vi "Check for errors.vi"(8 "error in (no error)":errorcluster, 11 "System states in":T1) -> (0 "error out":errorcluster, 3 "System states out":T1)   [LabVIEW 2015]
uses:
  Type defs/System states.ctl
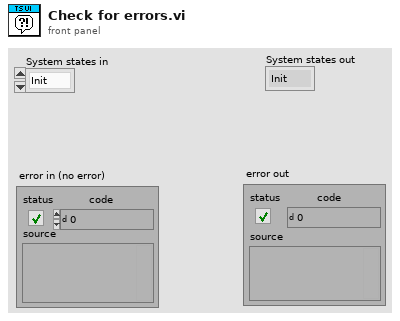
[diagram p1: front panel]
types:
  T1 = typedef "System states.ctl" = enum16{"Init", "Configure connections", "Register callbacks", "Start application", "Event handler", "Error handler", "Shutdown"}
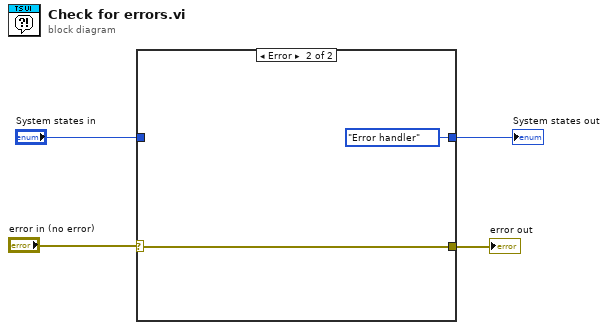
[diagram p0: block diagram]
diagram:
  n1 = case shown="Error" "error in (no error)" {
    selector: "error in (no error)" -> [w6 w8]
    tunnel: [w6 w8] -> w3
    tunnel: "System states in" -> [w5 _]
    tunnel: [w5 System_states."Error handler" ("System states in")] -> w1
    frame No Error {
    }
    frame Error {
    }
  }
  "System states out" <- w1
  "error out" <- w3
